vi "Close Instrument.vi"(8 "error in (no error)":errorcluster, 11 "instrument.Cryostation in":refnum<class "instrument.Cryostation.lvclass">) -> (0 "error out":errorcluster, 3 "instrument.Cryostation out":refnum<class "instrument.Cryostation.lvclass">)   [LabVIEW 2016, in "instrument.Cryostation.lvclass"]
uses:
  instrument.Cryostation.lvclass
  instrument.Cryostation.lvclass/instrument.Cryostation.ctl
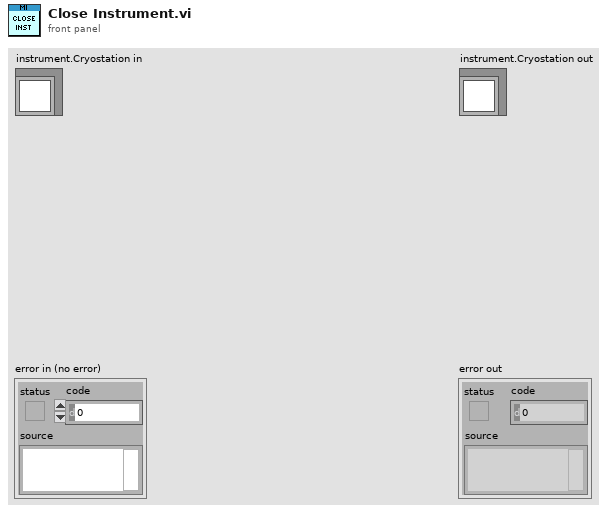
[diagram p1: front panel]
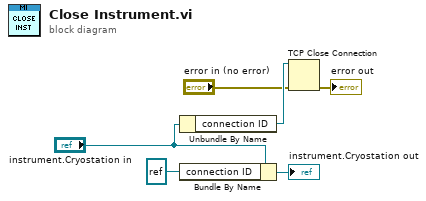
[diagram p0: block diagram]
diagram:
  n1 = Unbundle By Name("instrument.Cryostation in") -> ("connection ID"=w3:refnum<k5>)
  n2 = Bundle By Name(cluster="instrument.Cryostation in", "connection ID"=refnum<k5> refnum) -> (→"instrument.Cryostation out":refnum<class "instrument.Cryostation.lvclass">)
  n3 = TCP Close Connection(connection ID=w3, error in (no error)="error in (no error)") -> (error out=→"error out":errorcluster)  [unwired: 1 in, 1 out]
